vi "Escape Regex.vi"(7 "multiline? (F)":bool, 8 "error in (no error)":errorcluster, 11 "regex":string) -> (0 "error out":errorcluster, 3 "escaped regex":string)   [LabVIEW 2017]
doc: "Escapes regular expression string by inserting a backslash before the following characters: -()[]{}+?*.$^|,:#<!\\"
uses:
  <vilib>/regexp/Match Regular Expression.xnode
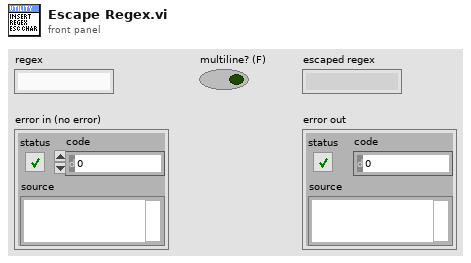
[diagram p1: front panel]
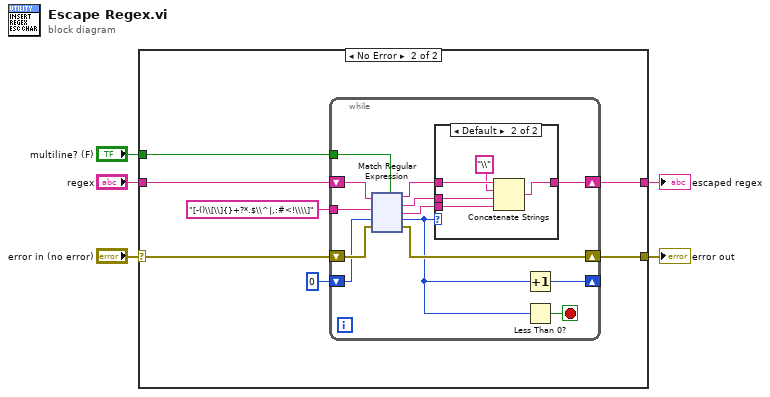
[diagram p0: block diagram]
diagram:
  n1 = case shown="No Error" "error in (no error)" {
    selector: "error in (no error)" -> [w7 w9]
    tunnel: "regex" -> [w6 w13]
    tunnel: [w6 w11] -> w4
    tunnel: [w7 w10] -> w2
    tunnel: "multiline? (F)" -> [_ w8]
    frame Error {
    }
    frame No Error {
      n2 = while {
        tunnel: "[-()\\[\\]{}+?*.$\\^|,:#<!\\\\]" ("search string") -> [w25]
        shift-right: [w20] -> w11
        shift-left: w13 -> [w24]
        shift-right: [w18] -> _
        shift-left: 0 ("offset past match") -> [w19]
        shift-right: [w27] -> w10
        shift-left: w9 -> [w26]
        tunnel: w8 -> [w15]
        stop <- w17 stop-if-true
        n3 = xnode "Match Regular Expression"("input string"=w24, "regular expression"=w25, "offset (0)"=w19, "error in"=w26, "multiline? (F)"=w15) -> ("before match"=w23:string, "whole match"=w22:string, "after match"=w21:string, "offset past match"=w16:i32, "error out"=w27:errorcluster)  [unwired: 1 in]
        n4 = case shown="Default" w16 {
          tunnel: w23 -> [w28 w33]
          tunnel: w22 -> [_ w32]
          tunnel: w21 -> [_ w31]
          tunnel: [w28 w29] -> w20
          frame ..-1 {
          }
          frame Default {
            n5 = Concatenate Strings(w33, "\\" ("string"), w32, w31) -> (w29:string)
          }
        }
        n6 = Increment(x=w16) -> (x+1=w18:i32)
        n7 = Less Than 0?(x=w16) -> (x < 0?=w17:bool)
      }
    }
  }
  "escaped regex" <- w4
  "error out" <- w2
